vi "Find RMS Velocity in_s .vi"(7 "Freq. Type":T1, 8 "error in (no error)":errorcluster, 9 "Sample Rate Hz":dbl, 10 "RPM":dbl, 11 "Y":dbl[](array[numeric])) -> (0 "error out":errorcluster, 3 "rms value":dbl)   [LabVIEW 2026, in "Acquisition.lvlib"]
uses:
  Acquisition.lvlib
  Controls/Frequency Type.ctl
  <vilib>/Analysis/3filter.llb/Filter Passband Type.ctl
  <vilib>/Analysis/5stat.llb/RMS (DBL).vi
  <vilib>/Analysis/3filter.llb/Butterworth Filter (DBL).vi
  <vilib>/Analysis/NI_AALBase.lvlib
  <vilib>/Analysis/NI_AALPro.lvlib
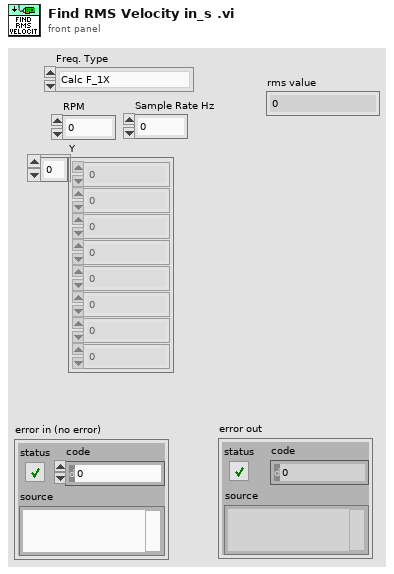
[diagram p1: front panel]
types:
  T1 = typedef "Frequency Type.ctl" = enum16{"Calc F_1X", "Calc F_cutoff"}
  T2 = typedef "NI_AALBase.lvlib/Filter Passband Type.ctl" = enum32{"Lowpass", "Highpass", "Bandpass", "Bandstop"}
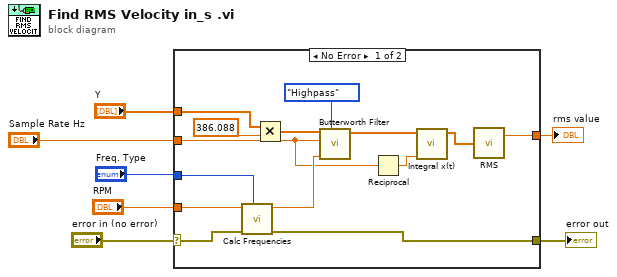
[diagram p0: block diagram]
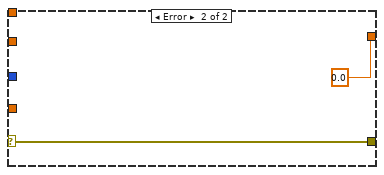
[diagram p2: hidden frame]
diagram:
  n1 = case shown="No Error" "error in (no error)" {
    selector: "error in (no error)" -> [w14 w23]
    tunnel: "Y" -> [w20 _]
    tunnel: [w13 w23] -> w5
    tunnel: [w15 0.0] -> w4
    tunnel: "Freq. Type" -> [w12 _]
    tunnel: "RPM" -> [w11 _]
    tunnel: "Sample Rate Hz" -> [w8 _]
    frame No Error {
      n2 = call "Calc Frequencies.vi"("Freq. Type"=w12, "error in (no error)"=w14, "RPM"=w11) -> ("error out"=w13:errorcluster, "f"=w10:dbl)  [unwired: 7 in]
      n3 = Multiply(x=w20, y=386.088) -> (x*y=w18:dbl[])
      n4 = call-poly <vilib>:"Butterworth Filter.vi"("filter type"=Filter_Passband_Type."Highpass", "low cutoff freq: fl"=w10, "sampling freq: fs"=w8, "X"=w18) -> ("Filtered X"=w17:dbl[])  [unwired: 4 in, 1 out]
      n5 = Reciprocal(x=w8) -> (1/x=w9:dbl)
      n6 = call <vilib>:"Integral x(t).vi"("dt"=w9, "X"=w17) -> ("Integral X"=w16:dbl[])  [unwired: 8 in, 1 out]
      n7 = call-poly <vilib>:"RMS.vi"("X"=w16) -> ("rms value"=w15:dbl)  [unwired: 1 out]
    }
    frame Error {
    }
  }
  "error out" <- w5
  "rms value" <- w4
